vi "Global 1.vi"() -> ()   [LabVIEW 2020]
panel:
  out "Flag":bool
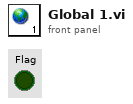
[diagram p1: front panel]
diagram:
